vi "record_vars.vi"(6 "save?":bool, 8 "error in":errorcluster, 9 "var1_values":dbl[](array[numeric]), 10 "var0_values":dbl[](array[numeric]), 11 "output":path[](array[path])) -> (0 "error out":errorcluster)   [LabVIEW 2017, in "tools.lvlib"]
uses:
  tools.lvlib
panel:
  out "v0 path":path
  out "v1 path":path
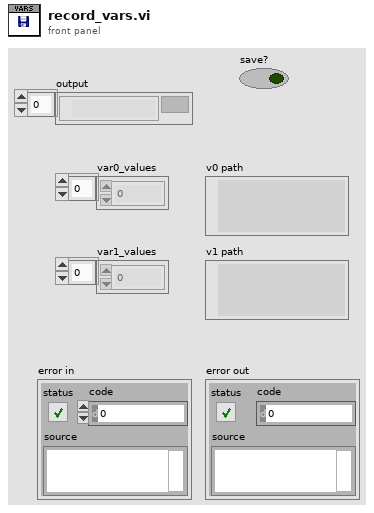
[diagram p1: front panel]
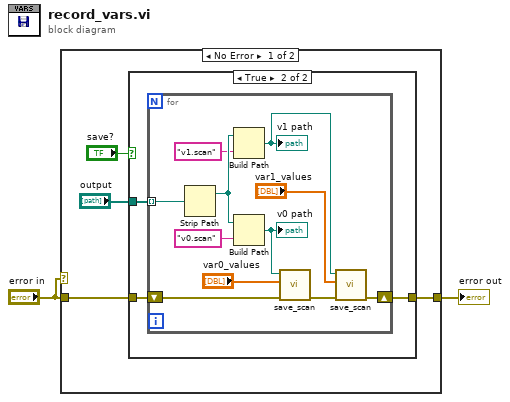
[diagram p0: block diagram]
diagram:
  n1 = case shown="No Error" "error in" {
    tunnel: "error in" -> [w4 w22]
    tunnel: [w3 w22] -> w2
    frame No Error {
      n2 = case shown="True" "save?" {
        tunnel: "output" -> [_ w10]
        tunnel: [w7 w9] -> w3
        tunnel: w4 -> [w7 w8]
        frame False {
        }
        frame True {
          n3 = for {
            tunnel: w10 -> [w21] mode=indexing
            shift-right: [w11] -> w9
            shift-left: w8 -> [w15]
            n4 = Strip Path(path=w21) -> (stripped path=w19:path)  [unwired: 1 out]
            n5 = Build Path(base path=w19, name or relative path="v1.scan") -> (appended path=w14:path)
            "v1 path" <- w14
            n6 = Build Path(base path=w19, name or relative path="v0.scan") -> (appended path=w17:path)
            "v0 path" <- w17
            n7 = call "save_scan.vi"("error in"=w15, "values in"="var0_values", "path"=w17) -> ("error out"=w13:errorcluster)  [unwired: 8 in]
            n8 = call "save_scan.vi"("error in"=w13, "values in"="var1_values", "path"=w14) -> ("error out"=w11:errorcluster)  [unwired: 8 in]
          }
        }
      }
    }
    frame Error {
    }
  }
  "error out" <- w2
